vi "GetDeviceAddress.vi"(8 "error in (no error)":errorcluster, 10 "DeviceKey In":string, 11 "CmdLib In":refnum<k24>) -> (0 "error out":errorcluster, 1 "Device Address":i32, 2 "DeviceKey Out":string, 3 "CmdLib Out":refnum<k24>)   [LabVIEW 2019]
uses:
  C:/Users/jyxks/OneDrive/Documents/Program Files/New Focus/New Focus Picomotor Application/Samples/LabVIEW/Model 8742/LabVIEW 2009/CmdLib.dll
  Program Files/New Focus/New Focus Picomotor Application/Samples/LabVIEW/Model 8742/LabVIEW 2009/CmdLib.dll
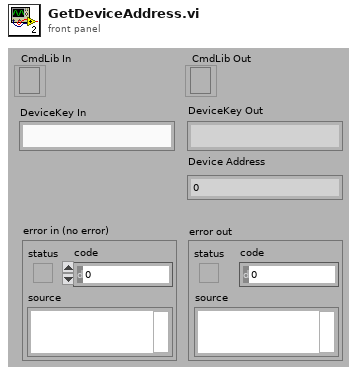
[diagram p1: front panel]
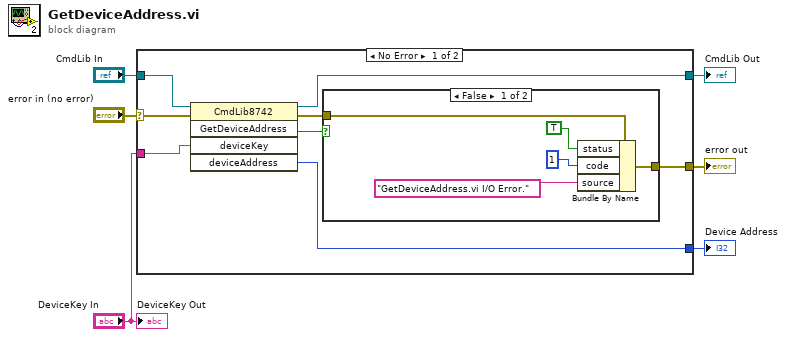
[diagram p0: block diagram]
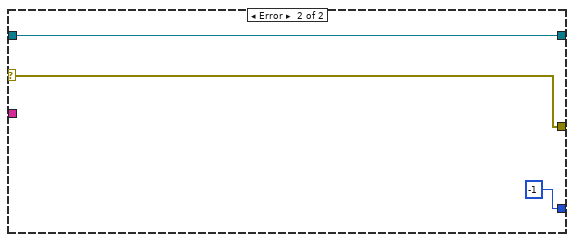
[diagram p3: hidden frame]
diagram:
  n1 = case shown="No Error" "error in (no error)" {
    selector: "error in (no error)" -> [w11 w22]
    tunnel: "CmdLib In" -> [w14 w23]
    tunnel: [w13 w23] -> w5
    tunnel: "DeviceKey In" -> [w12 _]
    tunnel: [w8 w22] -> w2
    tunnel: [w7 -1] -> w1
    frame No Error {
      n2 = invoke class="CmdLib8742" method="GetDeviceAddress"(reference=w14, error in=w11, "deviceKey"=w12) -> (reference out=w13:refnum<k24>, error out=w9:errorcluster, "GetDeviceAddress"=w10:bool, "deviceAddress"=w7:i32)  [unwired: 2 in, 1 out]
      n3 = case shown="False" w10 {
        tunnel: w9 -> [w19 w20]
        tunnel: [w18 w20] -> w8
        frame False {
          n4 = Bundle By Name(cluster=w19, "status"=TRUE, "code"=1, "source"="GetDeviceAddress.vi I/O Error.") -> (w18:errorcluster)
        }
        frame True {
        }
      }
    }
    frame Error {
    }
  }
  "error out" <- w2
  "CmdLib Out" <- w5
  "Device Address" <- w1
  "DeviceKey Out" <- "DeviceKey In"
